vi "Configure Raster Scan Parameters.vi"(7 "Trigger Delay to Galvo":u16, 8 "error in":errorcluster, 9 "Y Trigs Info":T1, 10 "X Trigs Info":T2, 11 "FPGA VI Reference In":refnum<k20>) -> (0 "error out":errorcluster, 3 "FPGA VI Reference Out":refnum<k20>)   [LabVIEW 2011]
uses:
  <vilib>/Utility/error.llb/Error Cluster From Error Code.vi
  <vilib>/rvi/errors/niLvFpgaAdjustHostInterfaceError.vi
  <vilib>/rvi/interface/nirviReadWriteControl/nirviReadWriteControl.xnode
  NiFpgaLv.dll
  <vilib>/rvi/interface/Simulation/niFpgaSimulationCallBeginRW.vi
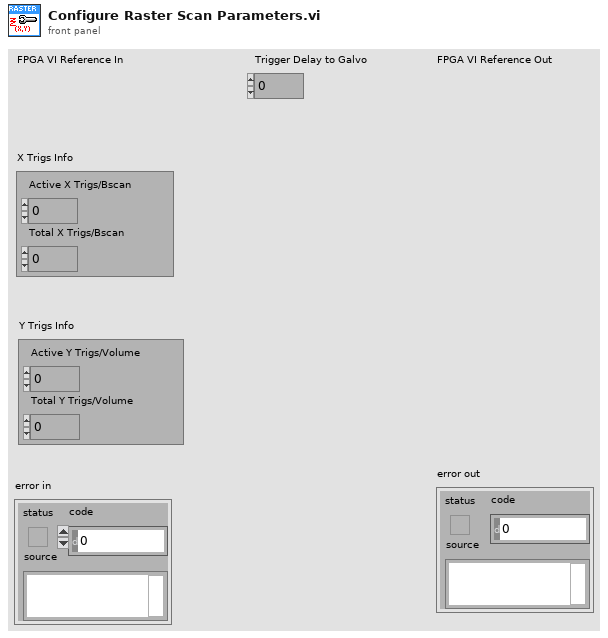
[diagram p1: front panel]
types:
  T1 = cluster{"Active Y Trigs/Volume":u16, "Total Y Trigs/Volume":u16}
  T2 = cluster{"Active X Trigs/Bscan ":u16, "Total X Trigs/Bscan":u16}
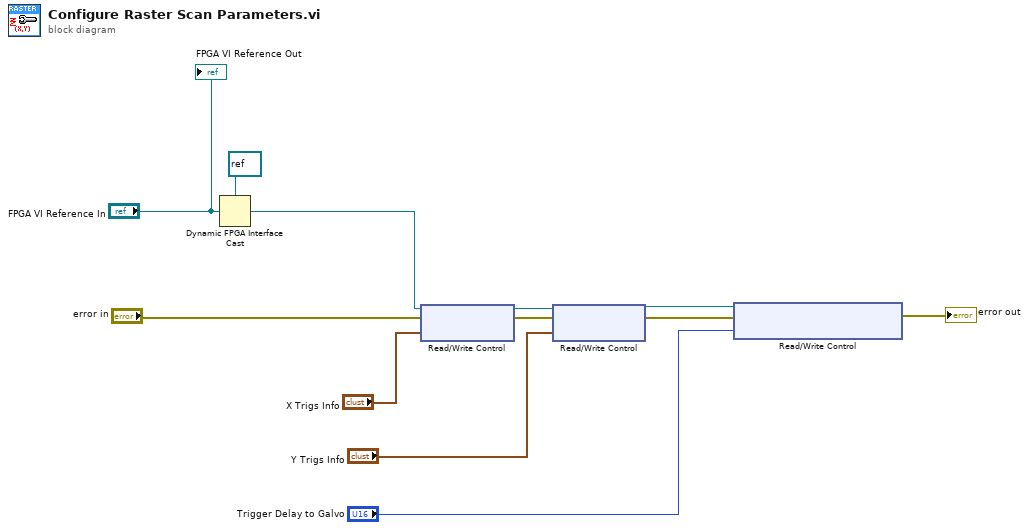
[diagram p0: block diagram]
diagram:
  n1 = Dynamic FPGA Interface Cast(Session In=refnum<k20> refnum ("Type"), Type="FPGA VI Reference In") -> (Session Out=w10:refnum<k20>)
  n2 = xnode "Read/Write Control"("FPGA VI Reference In"=w10, "error in"="error in", "X Trigs Info"="X Trigs Info") -> ("FPGA VI Reference Out"=w8:refnum<k20>, "error out"=w7:errorcluster)
  n3 = xnode "Read/Write Control"("FPGA VI Reference In"=w8, "error in"=w7, "Y Trigs Info"="Y Trigs Info") -> ("FPGA VI Reference Out"=w6:refnum<k20>, "error out"=w5:errorcluster)
  n4 = xnode "Read/Write Control"("FPGA VI Reference In"=w6, "error in"=w5, "Trigger Delay to Galvo"="Trigger Delay to Galvo") -> ("error out"=→"error out":errorcluster)  [unwired: 1 out]
  "FPGA VI Reference Out" <- "FPGA VI Reference In"
